vi "CliGetPlcDateTime.vi"(0 "ref in":u64, 11 "error in (no error)":errorcluster) -> (4 "ref out":u64, 6 "Result":i32, 8 "DateTime":timestamp, 15 "error out":errorcluster)   [LabVIEW 2018, in "Snap7.lvlib"]
uses:
  Snap7.lvlib
  windows/lv_snap7.dll
panel:
  in  "var TimeStamp":timestamp
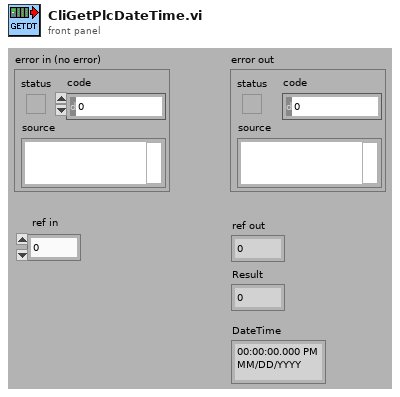
[diagram p1: front panel]
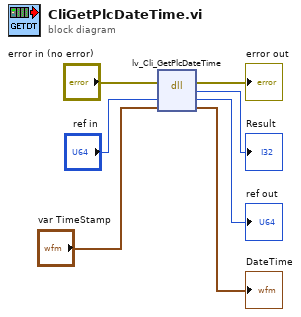
[diagram p0: block diagram]
diagram:
  n1 = dll-call lib="PTH2iabs D项目Feng恒隆项目Labview性能试验台SourcesSnap7libwindowslv_snap7.dll" fn="lv_Cli_GetPlcDateTime"(error in="error in (no error)", "Client"="ref in", "var_timestamp"="var TimeStamp") -> (error out=→"error out":errorcluster, "return type"=→"Result":i32, "Client"=→"ref out":u64, "var_timestamp"=→"DateTime":timestamp)  [unwired: 2 in, 1 out]
